vi "CC Subsystem Status FG.vi"(7 "Action":T2, 8 "error in (no error)":errorcluster, 10 "Status":T1, 11 "Subsystem Name":string) -> (0 "error out":errorcluster, 2 "status out":T1)   [LabVIEW 2024]
uses:
  typedefs/CC enum Status FG Action.ctl
  typedefs/CC enum Subsystem Status.ctl
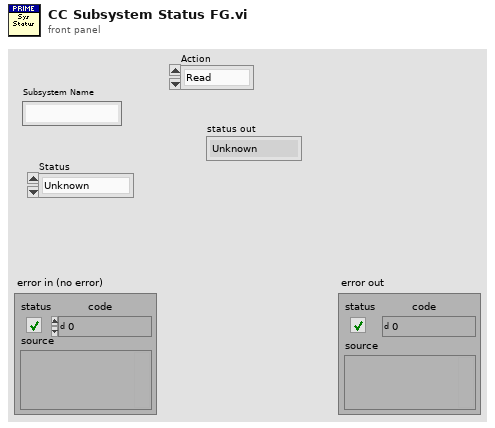
[diagram p1: front panel]
types:
  T1 = typedef "CC enum Subsystem Status.ctl" = enum16{"Unknown", "Ready", "Error"}
  T2 = typedef "CC enum Status FG Action.ctl" = enum16{"Read", "Write", "Init"}
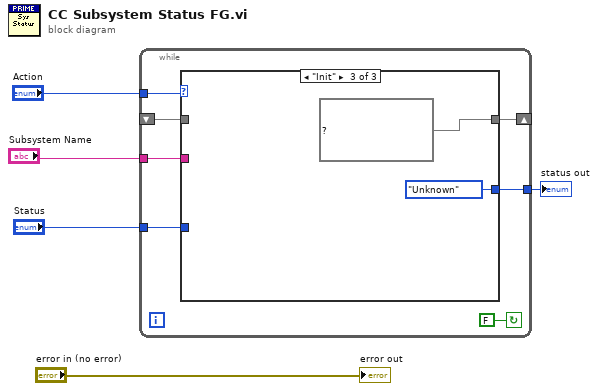
[diagram p0: block diagram]
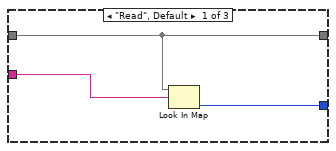
[diagram p2: hidden frame]
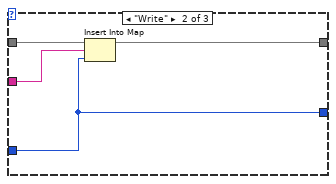
[diagram p3: hidden frame]
diagram:
  n1 = while {
    tunnel: "Action" -> [w12]
    shift-right: [w8] -> _
    shift-left: _ -> [w7]
    tunnel: "Subsystem Name" -> [w10]
    tunnel: "Status" -> [w9]
    tunnel: [w6] -> w1
    stop <- FALSE continue-if-true
    n2 = case shown="\"Init\"" w12 {
      tunnel: w10 -> [w14 w18 _]
      tunnel: w9 -> [_ w17 _]
      tunnel: [w15 w16 map{string, T1} {} ("map")] -> w8
      tunnel: w7 -> [w15 w19 _]
      tunnel: [w13 w17 CC_enum_Subsystem_Status."Unknown" ("Status")] -> w6
      frame "Read", Default {
        n3 = Look In Map(map=w15, key=w14) -> (value=w13:T1)  [unwired: 1 in, 1 out]
      }
      frame "Write" {
        n4 = Insert Into Map(map in=w19, key=w18, value=w17) -> (map out=w16:map{string, T1})  [unwired: 2 out]
      }
      frame "Init" {
      }
    }
  }
  "status out" <- w1
  "error out" <- "error in (no error)"
